vi "Record Path.vi"(9 "Record Path":bool) -> ()   [LabVIEW 2020]
uses:
  Framework/Robot Global Data.vi
  <vilib>/Analysis/Matrix/Numeric/Conversions/Matrix To Array - RM.vi
  <vilib>/Utility/file.llb/Write Delimited Spreadsheet (DBL).vi
  <vilib>/Analysis/Matrix/NI_Matrix.lvlib
panel:
  out "path":path
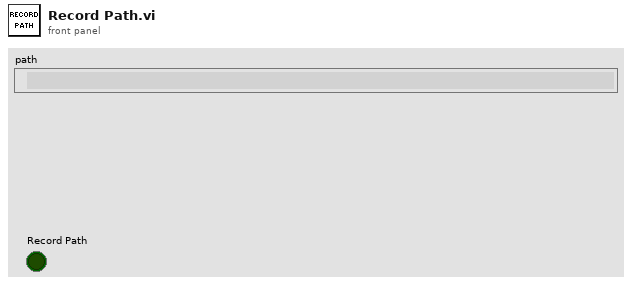
[diagram p1: front panel]
types:
  T1 = typedef "NI_Matrix.lvlib/RealMatrix.ctl" = dbl[][]
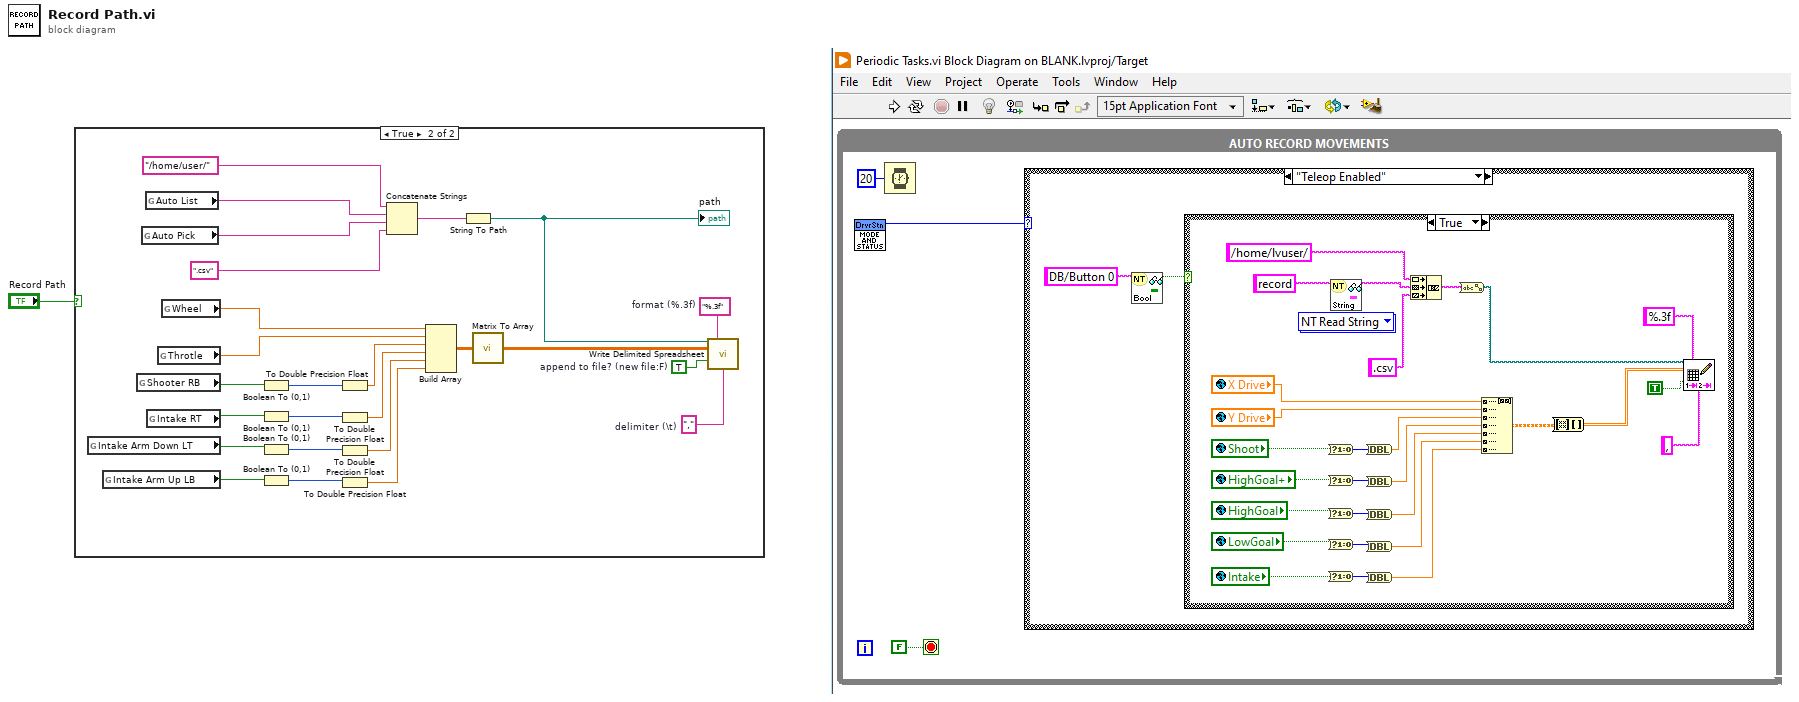
[diagram p0: block diagram]
diagram:
  n1 = case shown="True" "Record Path" {
    frame False {
    }
    frame True {
      w15 = TRUE  # append to file? (new file:F)
      w16 = "%.3f"  # format (%.3f)
      w11 = ","  # delimiter (\t)
      n2 = global read "Robot Global Data.vi" "Intake Arm Down LT"() -> (w6:bool)
      n3 = global read "Robot Global Data.vi" "Intake Arm Up LB"() -> (w5:bool)
      n4 = global read "Robot Global Data.vi" "Shooter RB"() -> (w8:bool)
      n5 = global read "Robot Global Data.vi" "Auto Pick"() -> (w3:string)
      n6 = global read "Robot Global Data.vi" "Auto List"() -> (w4:string)
      n7 = global read "Robot Global Data.vi" "Intake RT"() -> (w7:bool)
      n8 = global read "Robot Global Data.vi" "Throtle"() -> (w9:dbl)
      n9 = global read "Robot Global Data.vi" "Wheel"() -> (w10:dbl)
      n10 = Boolean To (0,1)(Boolean=w8) -> (0, 1=w24:i16)
      n11 = Boolean To (0,1)(Boolean=w7) -> (0, 1=w23:i16)
      n12 = Boolean To (0,1)(Boolean=w6) -> (0, 1=w22:i16)
      n13 = Boolean To (0,1)(Boolean=w5) -> (0, 1=w21:i16)
      n14 = To Double Precision Float(number=w24) -> (double precision float=w20:dbl)
      n15 = To Double Precision Float(number=w23) -> (double precision float=w19:dbl)
      n16 = To Double Precision Float(number=w22) -> (double precision float=w18:dbl)
      n17 = To Double Precision Float(number=w21) -> (double precision float=w17:dbl)
      n18 = Concatenate Strings("/home/user/", w4, w3, ".csv") -> (w12:string)
      n19 = Build Array(w10, w9, w20, w19, w18, w17) -> (w26:T1)
      n20 = String To Path(string=w12) -> (path=w2:path)
      "path" <- w2
      n21 = call-poly <vilib>:"Matrix To Array.vi"("Real Matrix"=w26) -> ("Real 2D Array"=w25:dbl[][])
      n22 = call-poly <vilib>:"Write Delimited Spreadsheet.vi"("file path (dialog if empty)"=w2, "format (%.3f)"=w16, "2D data"=w25, "append to file? (new file:F)"=w15, "delimiter (\\t)"=w11) -> ()  [unwired: 9 in, 2 out]
    }
  }
